vi "Convert RPC Error to LabVIEW Error.vi"(9 "JSON Value in":variant, 11 "RPC Error Code":i32) -> (2 "error out":errorcluster)   [LabVIEW 2020, in "JSON-RPC Lib.lvlib" / "JSONRPC Client.lvclass"]
uses:
  JSONRPC Client.lvclass
  Variant Data Manipulation/Variant Data Manipulation.lvlib
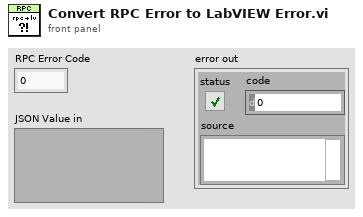
[diagram p1: front panel]
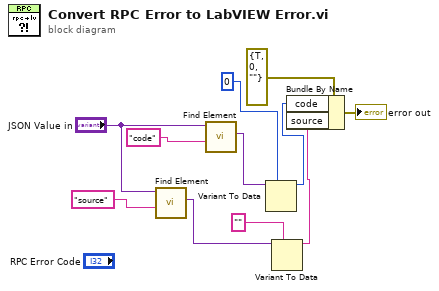
[diagram p0: block diagram]
diagram:
  n1 = call "Find Element.vi"("Name"="source" ("key"), "Variant (Cluster) in"="JSON Value in") -> ("element"=w3:variant)  [unwired: 5 in, 4 out]
  n2 = call "Find Element.vi"("Name"="code" ("Parameter Name"), "Variant (Cluster) in"="JSON Value in") -> ("element"=w6:variant)  [unwired: 5 in, 4 out]
  n3 = Variant To Data(type=0 ("code"), Variant=w6) -> (data=w5:i32)  [unwired: 1 in, 1 out]
  n4 = Variant To Data(type="" ("source"), Variant=w3) -> (data=w1:string)  [unwired: 1 in, 1 out]
  n5 = Bundle By Name(cluster=errorcluster {"status"=TRUE, "code"=0, "source"=""} ("error constant"), "code"=w5, "source"=w1) -> (→"error out":errorcluster)
